vi "Lin_Rohner_lab2A_question4.vi"() -> ()   [LabVIEW 2019]
uses:
  <vilib>/Platform/TimedLoop/XDataNode/timing_clust.ctl
  <vilib>/Platform/TimedLoop/XDataNode/nitl_modes.ctl
  <vilib>/Platform/TimedLoop/XDataNode/wakeup.ctl
  <vilib>/Analysis/3filter.llb/Filter Passband Type.ctl
  <vilib>/DAQmx/read.llb/DAQmx Read (Analog DBL 1Chan 1Samp).vi
  <vilib>/DAQmx/create/channels.llb/DAQmx Create Channel (AI-Voltage-Basic).vi
  <vilib>/DAQmx/miscellaneous.llb/DAQmx Fill In Error Info.vi
  <vilib>/platform/TimedLoop/XDataNode/XDataNode.xnode
  <vilib>/Platform/TimedLoop/XDataNode/XDNodeRunTimeDep.lvlib
  <vilib>/Analysis/NI_AALBase.lvlib
  <vilib>/ptbypt/NI_PtbyPt.lvlib
panel:
  out "Iteration":i32
  out "Raw Position":dbl
  out "Raw Position Graph":dbl(graph)
  out "Raw Acceleration":dbl
  out "Raw Velocity":dbl
  out "Filtered Velocity":dbl
  out "Filtered Velocity Graph":dbl(graph)
  in  "low cutoff freq:  Velocity":dbl=0.125 format="%0.3f"
  out "Filtered Acceleration":dbl
  out "Filtered Acceleration Graph":dbl(graph)
  in  "low cutoff freq: Acceleration":dbl=0.125 format="%0.3f"
  out "Raw Acceleration Graph":dbl(graph)
  out "Raw Veloctiy Graph":dbl(graph)
  in  "low cutoff freq: Position":dbl=0.125 format="%0.3f"
  out "Filtered Postion Graph":dbl(graph)
  out "Filtered Position":dbl
  in  "STOP":bool
  out "Position":dbl(knob) scale=-32.5..32.5
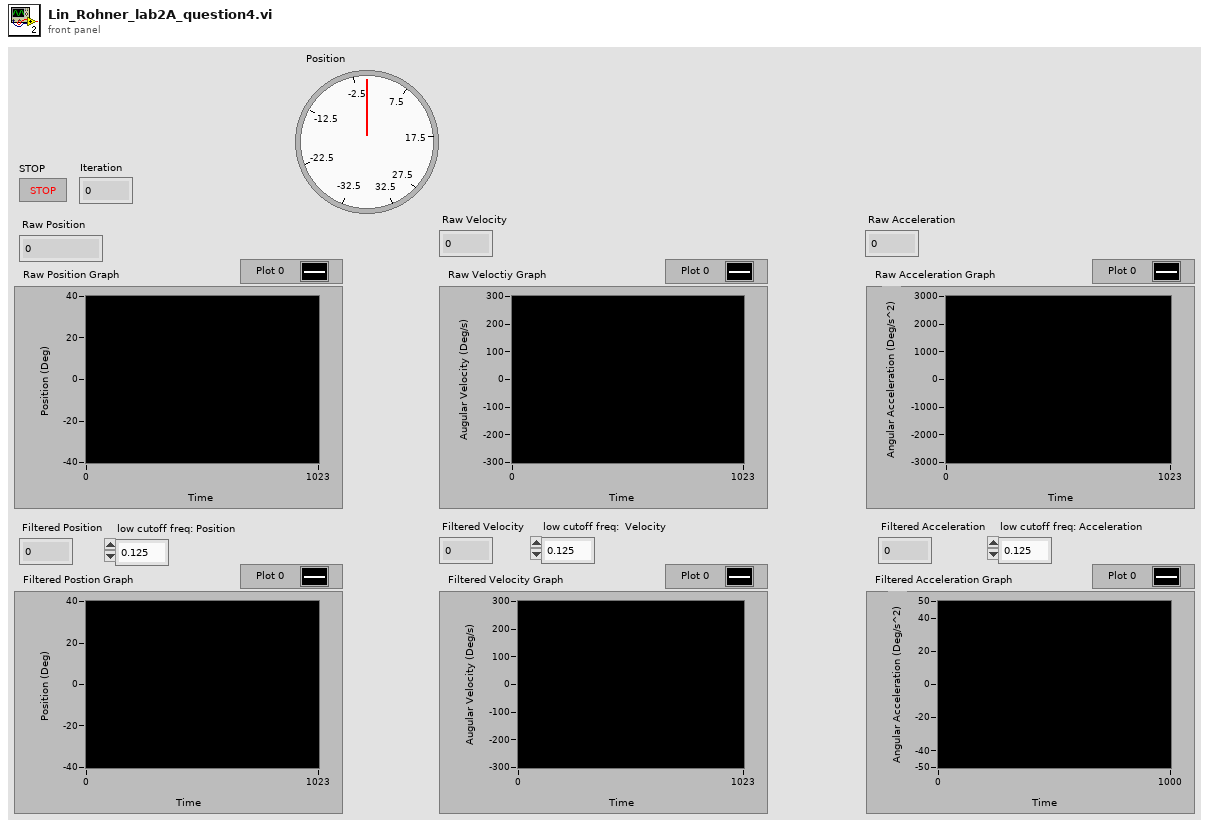
[diagram p1: front panel]
types:
  T1 = typedef "NI_AALBase.lvlib/Filter Passband Type.ctl" = enum32{"Lowpass", "Highpass", "Bandpass", "Bandstop"}
  T2 = typedef "XDNodeRunTimeDep.lvlib/timing_clust.ctl" = cluster{"Expected End [f-1]":u64, "Actual End [f-1]":u64, "Finished Late? [f-1]":bool, "Expected End [i-1]":u64, "Actual End [i-1]":u64, "Finished Late? [i-1]":bool, "Expected Start [i]":u64, "Actual Start [i]":u64, "Expected Start [f]":u64, "Actual Start [f]":u64, "Source Name":string, "Structure Name":string, "Period":i64, "Deadline":i64, "Offset":i64, "Start":i64, "Priority":i32, "Timeout":i32, "Mode":T3, "Wakeup Reason":T4, "Error":errorcluster, "Source Type":string, "Secondary Source Type":string, "Global End Time":u64, "Global Start Time":u64, "Frame Duration":u64, "Iteration Duration":u64, "Assigned CPU":i32, "I/O Scan Engine Mode":u32}
  T3 = typedef "XDNodeRunTimeDep.lvlib/nitl_modes.ctl" = enum32{"No Change", "Process missed periods, maintain original phase", "Discard missed periods, maintain original phase", "Process missed periods, ignore original phase", "Discard missed periods, ignore original phase"}
  T4 = typedef "XDNodeRunTimeDep.lvlib/wakeup.ctl" = enum32{"Normal", "Aborted", "Asynchronous wakeup", "Timing source error", "Timed loop error", "Timeout"}
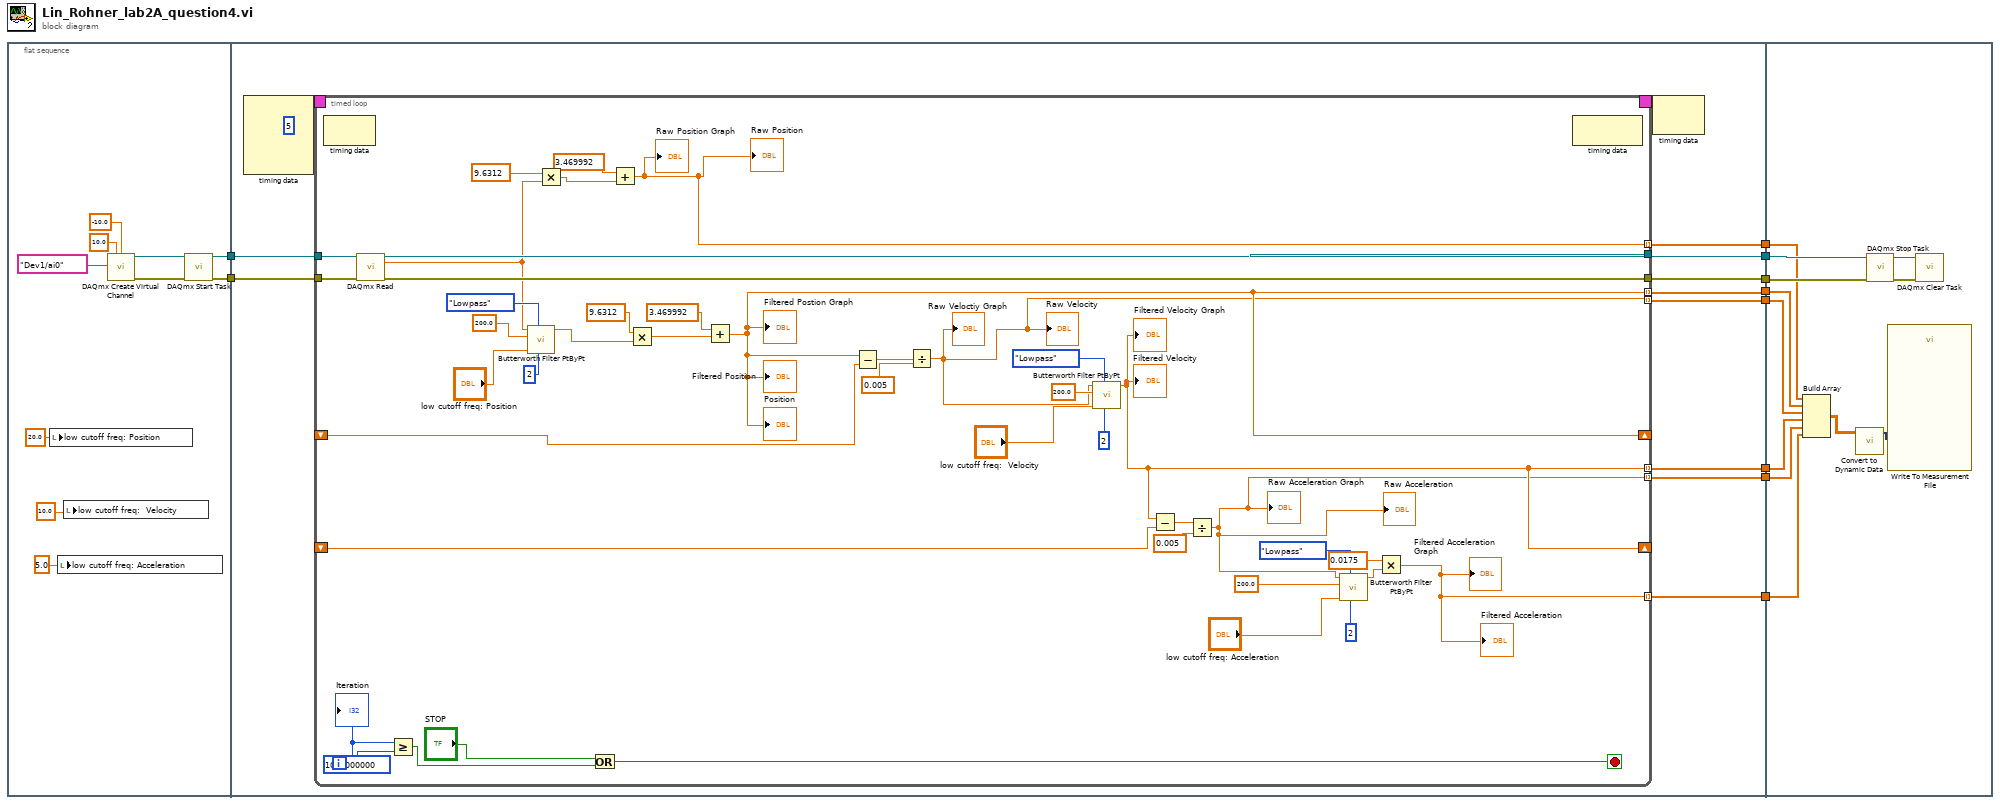
[diagram p0: block diagram]
diagram:
  n1 = flat-sequence {
    tunnel: [w16] -> w10
    tunnel: [w14] -> w9
    tunnel: w10 -> [w31]
    tunnel: [w30] -> w8
    tunnel: w9 -> [w29]
    tunnel: [w27] -> w7
    tunnel: [w26] -> w6
    tunnel: [w25] -> w5
    tunnel: [w24] -> w4
    tunnel: [w23] -> w3
    tunnel: [w22] -> w2
    tunnel: [w21] -> w1
    tunnel: w8 -> [w94]
    tunnel: w7 -> [w92]
    tunnel: w6 -> [w88]
    tunnel: w5 -> [w86]
    tunnel: w4 -> [w84]
    tunnel: w3 -> [w89]
    tunnel: w2 -> [w87]
    tunnel: w1 -> [w85]
    frame #0 {
      n2 = local write "low cutoff freq: Position"(20.0 ("low cutoff freq: Position")) -> ()
      n3 = local write "low cutoff freq: Acceleration"(5.0 ("low cutoff freq: Acceleration")) -> ()
      n4 = local write "low cutoff freq:  Velocity"(10.0 ("low cutoff freq:  Velocity")) -> ()
      n5 = call-poly <vilib>:"DAQmx Create Virtual Channel.vi"("maximum value"=10.0, "minimum value"=-10.0, "physical channels"=tag "Dev1/ai0") -> ("task out"=w15:refnum<k21>, "error out"=w17:errorcluster)  [unwired: 11 in]
      n6 = call <vilib>:"DAQmx Start Task.vi"("task/channels in"=w15, "error in"=w17) -> ("task out"=w14:refnum<k21>, "error out"=w16:errorcluster)  [unwired: 12 in]
    }
    frame #1 {
      n7 = node-c288(i64 5 ("Period")) -> (w33:T2)  [unwired: 3 in]
      n8 = timed-loop {
        timing: w33 -> [_]
        timing-out: [_] -> w32
        tunnel: w31 -> [w76]
        tunnel: [w75] -> w30
        tunnel: w29 -> [w70]
        tunnel: [w69] -> w27
        shift-right: [w41] -> _
        shift-left: _ -> [w47]
        shift-right: [w40] -> _
        shift-left: _ -> [w66]
        tunnel: [w41] -> w26 mode=indexing
        tunnel: [w40] -> w25 mode=indexing
        tunnel: [w34] -> w24 mode=indexing
        tunnel: [w39] -> w23 mode=indexing
        tunnel: [w38] -> w22 mode=indexing
        tunnel: [w37] -> w21 mode=indexing
        i -> [w45]
        stop <- w42 stop-if-true
        n9 = node-c288() -> ()  [unwired: 1 in, 1 out]
        n10 = call-poly <vilib>:"DAQmx Read.vi"("task/channels in"=w70, "error in"=w76) -> ("task out"=w69:refnum<k21>, "data"=w52:dbl, "error out"=w75:errorcluster)  [unwired: 11 in]
        n11 = Greater Or Equal?(x=w45, y=1000000000) -> (x >= y?=w46:bool)
        n12 = call <vilib>:"Butterworth Filter PtByPt.vi"("order"=2, "filter type"=Filter_Passband_Type."Lowpass", "low cutoff freq: fl"="low cutoff freq: Position", "sampling freq: fs"=200.0, "x"=w52) -> ("Filtered x"=w48:dbl)  [unwired: 4 in, 1 out]
        n13 = Multiply(x=9.6312, y=w52) -> (x*y=w54:dbl)
        n14 = Or(x="STOP", y=w46) -> (x .or. y?=w42:bool)
        n15 = Add(x=3.469992, y=w54) -> (x+y=w39:dbl)
        "Raw Position Graph" <- w39
        "Raw Position" <- w39
        n16 = Multiply(x=9.6312, y=w48) -> (x*y=w50:dbl)
        n17 = Add(x=3.469992, y=w50) -> (x+y=w41:dbl)
        "Filtered Postion Graph" <- w41
        "Filtered Position" <- w41
        "Position" <- w41
        n18 = Subtract(x=w41, y=w47) -> (x-y=w68:dbl)
        n19 = Divide(x=w68, y=0.005) -> (x/y=w38:dbl)
        "Raw Veloctiy Graph" <- w38
        "Raw Velocity" <- w38
        n20 = call <vilib>:"Butterworth Filter PtByPt.vi"("order"=2, "filter type"=Filter_Passband_Type."Lowpass", "low cutoff freq: fl"="low cutoff freq:  Velocity", "sampling freq: fs"=200.0, "x"=w38) -> ("Filtered x"=w40:dbl)  [unwired: 4 in, 1 out]
        "Filtered Velocity Graph" <- w40
        "Filtered Velocity" <- w40
        n21 = Subtract(x=w40, y=w66) -> (x-y=w65:dbl)
        n22 = Divide(x=w65, y=0.005) -> (x/y=w37:dbl)
        "Raw Acceleration Graph" <- w37
        "Raw Acceleration" <- w37
        n23 = call <vilib>:"Butterworth Filter PtByPt.vi"("order"=2, "filter type"=Filter_Passband_Type."Lowpass", "low cutoff freq: fl"="low cutoff freq: Acceleration", "sampling freq: fs"=200.0, "x"=w37) -> ("Filtered x"=w36:dbl)  [unwired: 4 in, 1 out]
        n24 = Multiply(x=0.0175, y=w36) -> (x*y=w34:dbl)
        "Filtered Acceleration Graph" <- w34
        "Filtered Acceleration" <- w34
        n25 = node-c288() -> ()  [unwired: 1 in, 1 out]
        "Iteration" <- w45
      }
      n26 = node-c288(w32) -> ()  [unwired: 1 out]
    }
    frame #2 {
      n27 = Build Array(w89, w88, w87, w86, w85, w84) -> (w83:dbl[][])
      n28 = call "Convert to Dynamic Data"("2D Array"=w83) -> ("Dynamic Data Type"=w90:dynamicdata)  [unwired: 3 in]
      n29 = call <vilib>:"DAQmx Stop Task.vi"("task/channels in"=w92, "error in"=w94) -> ("task out"=w91:refnum<k21>, "error out"=w93:errorcluster)  [unwired: 12 in]
      n30 = call "Write To Measurement File"("Signals"=w90) -> ()  [unwired: 16 in, 3 out]
      n31 = call <vilib>:"DAQmx Clear Task.vi"("task in"=w91, "error in"=w93) -> ()  [unwired: 13 in, 1 out]
    }
  }
